vi "array to design info.vi"(8 "error in (no error)":errorcluster, 11 "Array from file":cluster{"Label.Text":string, "Value":variant}[](array[cluster])=[{"Label.Text"="Project Name", "Value"=variant(string "")}, {"Label.Text"="City", "Value"=variant(string "")}, {"Label.Text"="State", "Value"=variant(string "")}, {"Label.Text"="Country", "Value"=variant(string "")}, {"Label.Text"="Notes", "Value"=variant(string "")}, {"Label.Text"="Q.Plant", "Value"=variant(dbl[unit] 0.005)}, {"Label.Text"="W.SedBay", "Value"=variant(dbl[unit] 1.0)}, {"Label.Text"="W.MpWalkway", "Value"=variant(dbl[unit] 1.5)}, {"Label.Text"="T.PlantWall", "Value"=variant(dbl[unit] 0.15)}, {"Label.Text"="EN.PipeSpec", "Value"=variant(enum16{"Schedule Number 10", "Schedule number 30\n", "Schedule Number 40", "Schedule Number 80\n", "Schedule Number 120", "Schedule Number 160\n", "SDR 17\n", "SDR 21\n", "SDR 26\n", "SDR 32.5\n", "SDR 41\n"} enum."SDR 26\n")}, {"Label.Text"="EN.DrillSeries", "Value"=variant(enum16{"English", "Metric"} enum."English")}, {"Label.Text"="C.FcmDoseMax", "Value"=variant(dbl[unit] 0.08)}, {"Label.Text"="C.FcmAlum", "Value"=variant(dbl[unit] 240.0)}, {"Label.Text"="T.FlocBaffle", "Value"=variant(dbl[unit] 0.02)}, {"Label.Text"="EN.FcmTube", "Value"=variant(enum16{"English", "Metric"} enum."English")}, {"Label.Text"="Ti.StockMin", "Value"=variant(dbl[unit] 108000.0)}, {"Label.Text"="N.SedTanks", "Value"=variant(dbl 3.0)}, {"Label.Text"="N.SedBaysEst", "Value"=variant(dbl 1.0)}, {"Label.Text"="L.SedPlateSheet", "Value"=variant(dbl[unit] 3.0)}, {"Label.Text"="W.SedSlopePlate", "Value"=variant(dbl[unit] 0.3)}, {"Label.Text"="T.SedSlopePlate", "Value"=variant(dbl[unit] 0.3)}, {"Label.Text"="Ti.SludgeDrain", "Value"=variant(dbl[unit] 1800.0)}, {"Label.Text"="CP.Floc", "Value"=variant(dbl 110.0)}, {"Label.Text"="ED.SedInlet", "Value"=variant(dbl[unit] 0.0005)}, {"Label.Text"="ED.Floc", "Value"=variant(dbl[unit][] [0.006, 0.0005])}, {"Label.Text"="W.FlocChannelMin", "Value"=variant(dbl[unit] 0.45)}, {"Label.Text"="Pi.FlowManifold", "Value"=variant(dbl 0.8)}, {"Label.Text"="V.SedUpBod", "Value"=variant(dbl[unit] 0.0008101851851851852)}, {"Label.Text"="V.SedCBod", "Value"=variant(dbl[unit] 0.00011574074074074073)}]) -> (0 "error out":errorcluster, 2 "Design Inputs":T2={"Q.Plant"=0.005, "C.CoagDoseMax"=0.01, "C.CoagStock"=0.015, "Ti.CoagStock"=0.0015, "EN.DrillSeries"=enum."English", "EN.TubeSeries"=enum."English", "N.SedTanks"=10.0, "N.SedBaysEst"=240.0, "W.SedPlate"=0.02, "L.SedPlateSheet"=0.0, "T.SedPlate"=388800000.0, "T.PlantWall"=0.03, "H.FlocOption"=0.01, "T.FlocBaffleRigidH"=0.03, "T.ConcreteMin"=0.3, "T.SedWeir"=0.3, "T.FlocBaffleRigidV"=108000.0} {"T.FlocBaffleRigidV" min=0.0 max=0.2 step=0.001 format="%#.1f"; "T.SedWeir" min=0.001 max=0.2 step=0.001 format="%#.1f"; "T.SedPlate" min=0.001 max=0.05 step=0.001 format="%#.1f"; "T.FlocBaffleRigidH" min=0.0 max=0.2 step=0.001 format="%#.1f"; "T.ConcreteMin" min=0.005 max=0.2 step=0.001 format="%#.1f"; "L.SedPlateSheet" min=0.3 max=8.0 step=0.01 format="%#.1f"; "N.SedBaysEst" min=1.0 max=20.0 step=1.0 format="%#.0f"; "N.SedTanks" min=1.0 max=20.0 step=1.0 format="%#.0f"; "Ti.CoagStock" min=43200.0 max=360000.0 step=3600.0 format="%#.1f"; "H.FlocOption" min=0.5 max=4.0 step=0.01 format="%#.2f"; "C.CoagStock" min=50.0 max=500.0 step=1.0 format="%#.0f"; "C.CoagDoseMax" min=0.03 max=0.2 step=0.005 format="%#.0f"; "Q.Plant" min=0.001 max=0.2 step=0.0001 format="%#.1f"; "T.PlantWall" min=0.05 max=0.5 step=0.001 format="%#.1f"; "W.SedPlate" min=0.5 max=3.0 step=0.001 format="%#.1f"}, 3 "Project Info":T1)   [LabVIEW 2015]
uses:
  Basic Inputs.ctl
  Project inputs.ctl
  AguaClara Library.lvlib
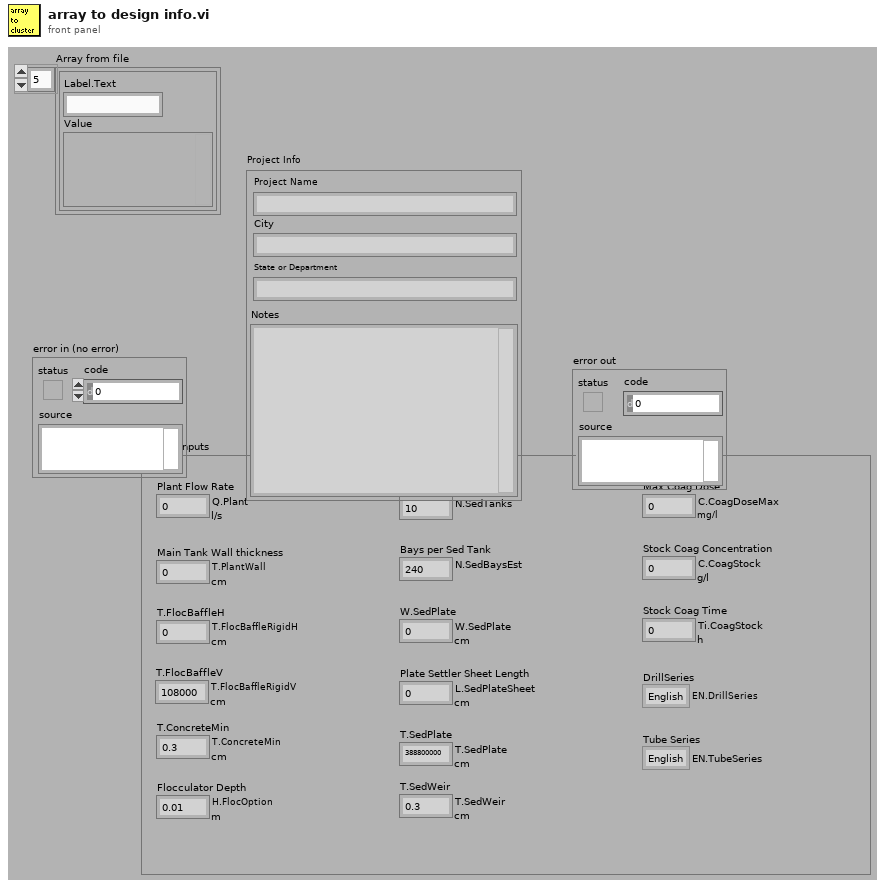
[diagram p1: front panel]
types:
  T1 = typedef "AguaClara Library.lvlib/Project inputs.ctl" = cluster{"Project Name":string, "City":string, "State":string, "Notes":string}
  T2 = typedef "AguaClara Library.lvlib/Basic Inputs.ctl" = cluster{"Q.Plant":dbl[unit], "C.CoagDoseMax":dbl[unit], "C.CoagStock":dbl[unit], "Ti.CoagStock":dbl[unit], "EN.DrillSeries":enum16{"English", "Metric"}, "EN.TubeSeries":enum16{"English", "Metric"}, "N.SedTanks":dbl, "N.SedBaysEst":dbl, "W.SedPlate":dbl[unit], "L.SedPlateSheet":dbl[unit], "T.SedPlate":dbl[unit], "T.PlantWall":dbl[unit], "H.FlocOption":dbl[unit], "T.FlocBaffleRigidH":dbl[unit], "T.ConcreteMin":dbl[unit], "T.SedWeir":dbl[unit], "T.FlocBaffleRigidV":dbl[unit]}
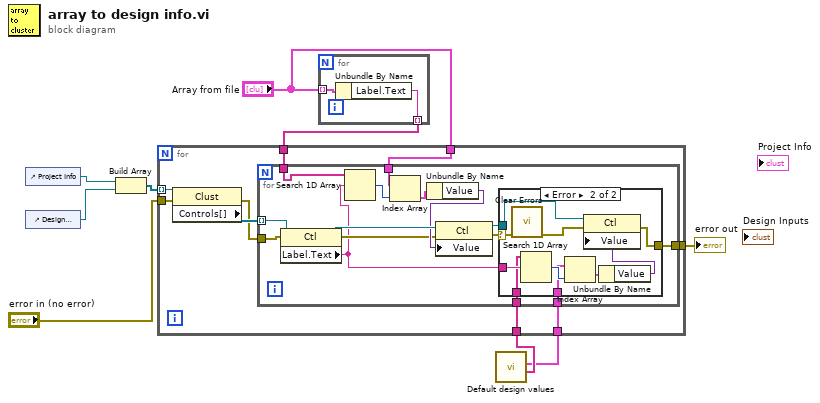
[diagram p0: block diagram]
diagram:
  n1 = control-ref of="Project Info"() -> (w9:refnum<vi>)
  n2 = control-ref of="Design Inputs"() -> (w8:refnum<vi>)
  n3 = Build Array(w9, w8) -> (w7:refnum<vi>[])
  n4 = for {
    tunnel: "Array from file" -> [w11] mode=indexing
    tunnel: [w10] -> w6 mode=indexing
    n5 = Unbundle By Name(w11) -> ("Label.Text"=w10:string)
  }
  n6 = call "Default design values.vi"() -> ("label array"=w2:string[], "Array to save"=w1:cluster{"Label.Text":string, "Value":variant}[])  [unwired: 9 in, 1 out]
  n7 = for {
    tunnel: w7 -> [w20] mode=indexing
    tunnel: w6 -> [w18]
    tunnel: "Array from file" -> [w17]
    tunnel: [w15] -> w4
    tunnel: "error in (no error)" -> [w14]
    tunnel: w2 -> [w13]
    tunnel: w1 -> [w12]
    n8 = property class="Clust"(reference=w20, error in=w14) -> (error out=w16:errorcluster, "Controls[]"=w19:refnum<vi>[])  [unwired: 1 out]
    n9 = for {
      tunnel: w19 -> [w35] mode=indexing
      tunnel: w18 -> [w34]
      tunnel: w17 -> [w33]
      tunnel: w16 -> [w28]
      tunnel: [w25] -> w15
      tunnel: w13 -> [w22]
      tunnel: w12 -> [w21]
      n10 = property class="Ctl"(reference=w35, error in=w28) -> (reference out=w31:refnum<vi>, error out=w27:errorcluster, "Label.Text"=w23:string)
      n11 = Search 1D Array(1D array=w34, element=w23) -> (index of element=w32:i32)  [unwired: 1 in]
      n12 = Index Array(array=w33, index=w32) -> (element=w30:cluster{"Label.Text":string, "Value":variant})
      n13 = Unbundle By Name(w30) -> ("Value"=w29:variant)
      n14 = property class="Ctl"(reference=w31, error in=w27, "Value"=w29) -> (reference out=w24:refnum<vi>, error out=w26:errorcluster)
      n15 = case shown="Error" w26 {
        selector: w26 -> [w36 w46]
        tunnel: [w36 w37] -> w25
        tunnel: w24 -> [_ w44]
        tunnel: w23 -> [_ w42]
        tunnel: w22 -> [_ w41]
        tunnel: w21 -> [_ w40]
        frame No Error {
        }
        frame Error {
          n16 = call <vilib>:"Clear Errors.vi"("error in (no error)"=w46) -> ("error out"=w45:errorcluster)  [unwired: 5 in, 1 out]
          n17 = Search 1D Array(1D array=w41, element=w42) -> (index of element=w43:i32)  [unwired: 1 in]
          n18 = Index Array(array=w40, index=w43) -> (element=w39:cluster{"Label.Text":string, "Value":variant})
          n19 = Unbundle By Name(w39) -> ("Value"=w38:variant)
          n20 = property class="Ctl"(reference=w44, error in=w45, "Value"=w38) -> (error out=w37:errorcluster)  [unwired: 1 out]
        }
      }
    }
  }
  "error out" <- w4
